vi "Initialize.vi"(7 "Serial Configuration":T1={"Baud Rate"=9600, "Parity"=0, "Data Bits"=8, "Stop Bits"=10, "Flow Control"=0} {"Flow Control" items=["None", "XON/XOFF", "RTS/CTS", "XON/XOFF & RTS/CTS", "DTR/DSR", "XON/XOFF & DTR/DSR"]; "Stop Bits" items=["1.0"=10, "1.5"=15, "2.0"=20]; "Data Bits" items=["7"=7, "8"=8]; "Parity" items=["None", "Odd", "Even", "Mark", "Space"]; "Baud Rate" items=["300"=300, "600"=600, "1200"=1200, "2400"=2400, "4800"=4800, "9600"=9600, "19200"=19200, "38400"=38400]}, 8 "error in (no error)":errorcluster, 9 "Reset (True)":bool=TRUE, 10 "ID Query (True)":bool=TRUE, 11 "VISA resource name":refnum<visa-resource-name>) -> (0 "error out":errorcluster, 3 "VISA resource name out":refnum<visa-resource-name>)   [LabVIEW 2014, in "Associated Research SC6540.lvlib"]
doc: "Establishes communication with the instrument and optionally performs an instrument identification query and/or an instrument reset. It also places the instrument in a default state needed for other instrument driver operations. Therefore, call this VI before calling other instrument driver VIs for this instrument. Generally, you need to call the Initialize VI only once at the beginning of an application."
uses:
  <instrlib>/Associated Research SC6540/Associated Research SC6540.lvlib
panel:
  # "(c) 2023  IKONIX Group.  ALL RIGHTS RESERVED."
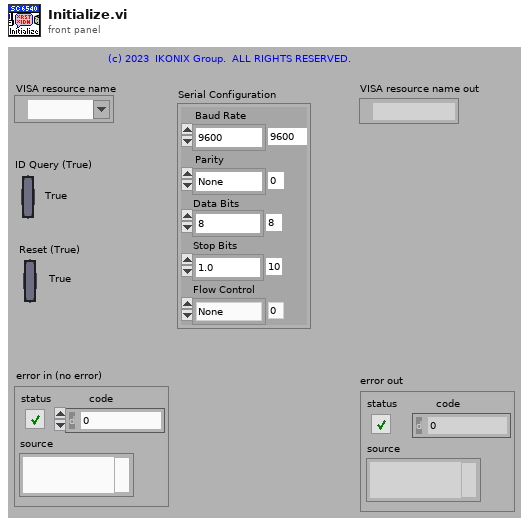
[diagram p1: front panel]
types:
  T1 = cluster{"Baud Rate":u32, "Parity":u16, "Data Bits":u16, "Stop Bits":u16, "Flow Control":u16}
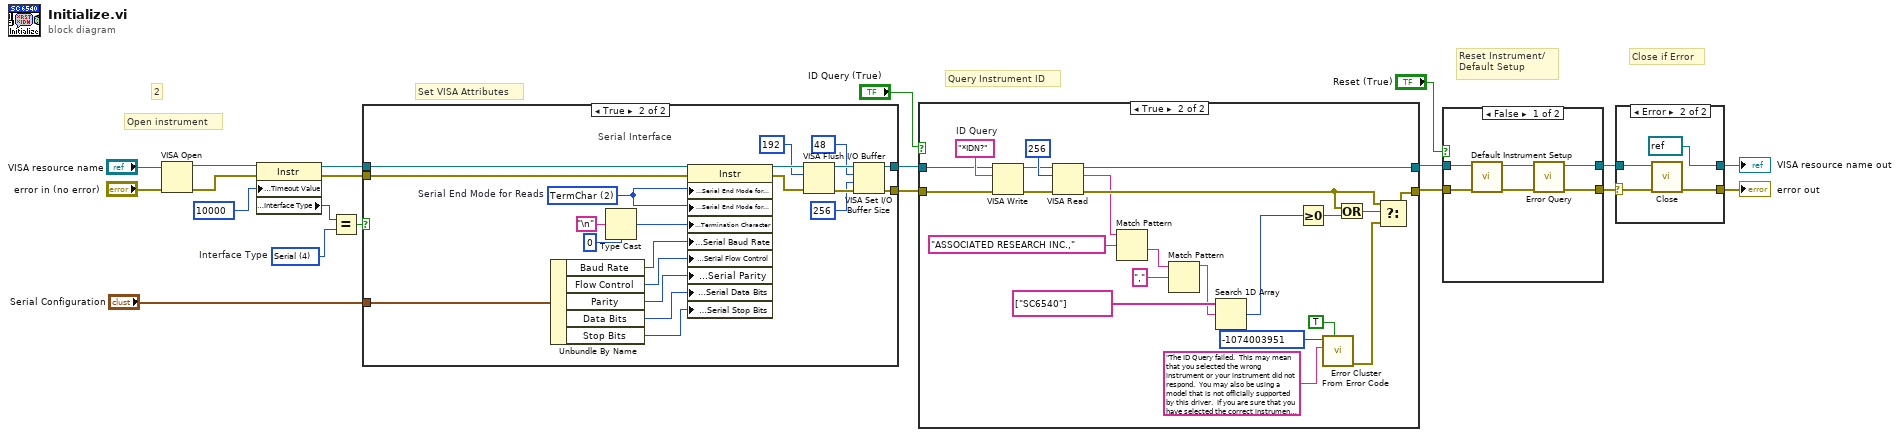
[diagram p0: block diagram]
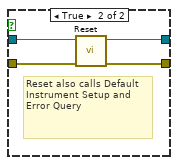
[diagram p4: hidden frame]
diagram:
  w6 = u16 4 items=["GPIB"=1, "VXI"=2, "GPIB-VXI"=3, "Serial"=4, "PXI"=5, "TCPIP"=6, "USB"=7]  # Interface Type
  # "2"
  # "Set VISA Attributes"
  # "Close if Error"
  # "Reset Instrument/\nDefault Setup"
  # "Query Instrument ID"
  # "Open instrument"
  n1 = VISA Open(error in (no error)="error in (no error)", VISA resource name="VISA resource name") -> (VISA resource name=w5:refnum<visa-resource-name>, error out=w2:errorcluster)  [unwired: 3 in]
  n2 = property on="属性节点" class="Instr"(reference=w5, error in=w2, "General Settings:Timeout Value"=u32 10000) -> (reference out=w9:refnum<visa-resource-name>, error out=w8:errorcluster, "Interface Information:Interface Type"=w11:u16)
  n3 = Equal?(x=w11, y=w6) -> (x = y?=w7:bool)
  n4 = case shown="True" w7 {
    tunnel: [w22 w41] -> w4
    tunnel: [w23 w38] -> w3
    tunnel: w9 -> [w22 w43]
    tunnel: w8 -> [w23 w44]
    tunnel: "Serial Configuration" -> [_ w24]
    frame False {
      # "GPIB Interface & Ethernet"
    }
    frame True {
      w31 = u16 2 items=["None", "LastBit", "TermChar"]  # Serial End Mode for Reads
      # "Serial Interface"
      n5 = Unbundle By Name(w24) -> ("Baud Rate"=w29:u32, "Flow Control"=w26:u16, "Parity"=w27:u16, "Data Bits"=w28:u16, "Stop Bits"=w25:u16)
      n6 = Type Cast(type=u8 0, x="\n" ("Line Feed Constant")) -> (*(type *) &x=w30:u8)
      n7 = property class="Instr"(reference=w43, error in=w44, "Serial Settings:Serial End Mode for Reads"=w31, "Serial Settings:Serial End Mode for Writes"=w31, "Message Based Settings:Termination Character"=w30, "Serial Settings:Serial Baud Rate"=w29, "Serial Settings:Serial Flow Control"=w26, "Serial Settings:Serial Parity"=w27, "Serial Settings:Serial Data Bits"=w28, "Serial Settings:Serial Stop Bits"=w25) -> (reference out=w37:refnum<visa-resource-name>, error out=w40:errorcluster)
      n8 = VISA Flush I/O Buffer(VISA resource name=w37, mask (16)=u16 192, error in (no error)=w40) -> (VISA resource name out=w42:refnum<visa-resource-name>, error out=w39:errorcluster)
      n9 = VISA Set I/O Buffer Size(VISA resource name=w42, mask (16)=u16 48, size (4096)=u32 256 ("size (0)"), error in (no error)=w39) -> (VISA resource name out=w41:refnum<visa-resource-name>, error out=w38:errorcluster)
    }
  }
  n10 = case shown="True" "ID Query (True)" {
    tunnel: [w45 w65] -> w20
    tunnel: [w46 w52] -> w21
    tunnel: w4 -> [w46 w55]
    tunnel: w3 -> [w45 w54]
    frame False {
    }
    frame True {
      w59 = "*IDN?"  # ID Query
      n11 = VISA Write(VISA resource name=w55, write buffer=w59, error in (no error)=w54) -> (VISA resource name out=w56:refnum<visa-resource-name>, error out=w57:errorcluster)  [unwired: 1 out]
      n12 = VISA Read(VISA resource name=w56, byte count=u32 256, error in (no error)=w57) -> (VISA resource name out=w52:refnum<visa-resource-name>, read buffer=w49:string, error out=w53:errorcluster)  [unwired: 1 out]
      n13 = Match Pattern(string=w49, regular expression="ASSOCIATED RESEARCH INC.," ("read buffer")) -> (after substring=w51:string)  [unwired: 1 in, 3 out]
      n14 = Match Pattern(string=w51, regular expression=",") -> (before substring=w48:string)  [unwired: 1 in, 3 out]
      n15 = Search 1D Array(1D array=string[] ["SC6540"] ("Instrument Models Supported"), element=w48) -> (index of element=w67:i32)  [unwired: 1 in]
      n16 = Greater Or Equal To 0?(x=w67) -> (x >= 0?=w66:bool)
      n17 = call <vilib>:"Error Cluster From Error Code.vi"("show call chain? (False)"=TRUE, "error message (\"\")"="The ID Query failed.  This may mean that you selected the wrong instrument or your instrument did not respond.  You may also be using a model that is not officially supported by this driver.  If you are sure that you have selected the correct instrument and it is responding, try disabling the ID Query." ("Source (VI Name)"), "error code (0)"=-1074003951 ("Code")) -> ("error out"=w60:errorcluster)  [unwired: 6 in]
      n18 = Or(x=w53, y=w66) -> (x .or. y?=w64:bool)
      n19 = Select(t=w53, s=w64, f=w60) -> (s? t:f=w65:errorcluster)
    }
  }
  n20 = case shown="False" "Reset (True)" {
    tunnel: w20 -> [w72 w75]
    tunnel: [w69 w78] -> w12
    tunnel: w21 -> [w74 w76]
    tunnel: [w71 w77] -> w17
    frame False {
      n21 = call <instrlib>:"Default Instrument Setup.vi"("error in (no error)"=w72, "VISA resource name"=w74) -> ("error out"=w70:errorcluster, "VISA resource name out"=w73:refnum<visa-resource-name>)  [unwired: 8 in]
      n22 = call <instrlib>:"Error Query.vi"("error in (no error)"=w70, "VISA resource name"=w73) -> ("error out"=w69:errorcluster, "VISA resource name out"=w71:refnum<visa-resource-name>)  [unwired: 6 in, 2 out]
    }
    frame True {
      # "Reset also calls Default Instrument Setup and Error Query"
      n23 = call <instrlib>:"Reset.vi"("error in (no error)"=w75, "VISA resource name"=w76) -> ("error out"=w78:errorcluster, "VISA resource name out"=w77:refnum<visa-resource-name>)  [unwired: 8 in]
    }
  }
  n24 = case shown="Error" w12 {
    selector: w12 -> [w79 w81]
    tunnel: w17 -> [w80 w83]
    tunnel: [w80 refnum<visa-resource-name> refnum ("VISA resource name out")] -> w16
    tunnel: [w79 w84] -> w15
    frame No Error {
    }
    frame Error {
      n25 = call <instrlib>:"Close.vi"("error in (no error)"=w81, "VISA resource name"=w83) -> ("error out"=w84:errorcluster)  [unwired: 9 in]
    }
  }
  "VISA resource name out" <- w16
  "error out" <- w15
